vi "A 正面结果分析.vi"(8 "Tbl引用句柄":refnum<vi>, 10 "列数":dbl, 11 "距离":string[][](array[string])) -> ()   [LabVIEW 2017]
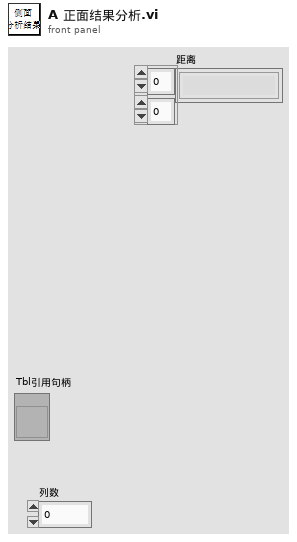
[diagram p1: front panel]
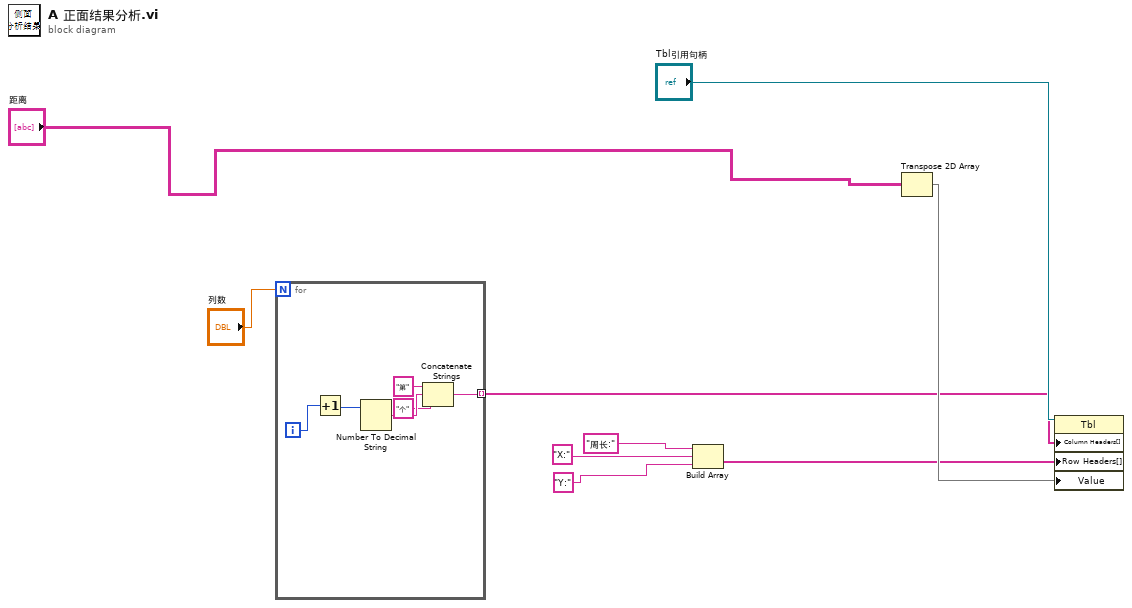
[diagram p0: block diagram]
diagram:
  n1 = for {
    N: "列数" -> [_]
    tunnel: [w10] -> w2 mode=indexing
    i -> [w15]
    n2 = Increment(x=w15) -> (x+1=w14:i32)
    n3 = Number To Decimal String(number=w14) -> (decimal integer string=w13:string)  [unwired: 1 in]
    n4 = Concatenate Strings("第" ("字符串"), w13, "个" ("字符串")) -> (w10:string)
  }
  n5 = Build Array("周长:", "X:", "Y:") -> (w4:string[])
  n6 = Transpose 2D Array(2D array="距离") -> (transposed array=w8:string[][])
  n7 = property class="Tbl"(reference="Tbl引用句柄", "Column Headers[]"=w2, "Row Headers[]"=w4, "Value"=w8) -> ()  [unwired: 1 in, 2 out]
